vi "Pickle.vi"(0 "variant":variant) -> (4 "pickle":string)   [LabVIEW 2015, in "LV Exceptions v1.lvlib"]
doc: "Alternative to 'Variant To Flattened String' function. The advantages are:\n* it returns only printable characters\n* complimentary function doesn't need 'type string' argument"
uses:
  LV Exceptions v1.lvlib
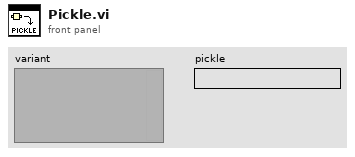
[diagram p1: front panel]
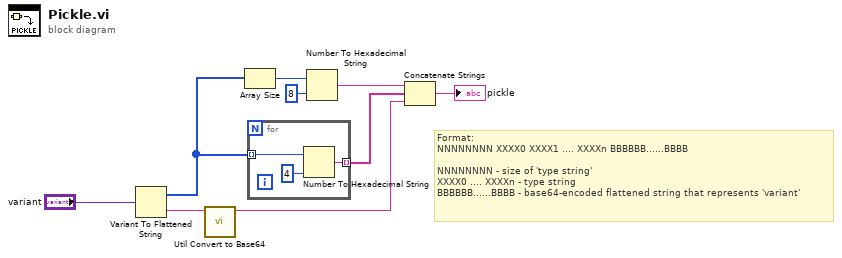
[diagram p0: block diagram]
diagram:
  # "Format:\nNNNNNNNN XXXX0 XXXX1 .... XXXXn BBBBBB......BBBB\n\nNNNNNNNN - size of 'type string'\nXXXX0 .... XXXXn - type string\nBBBBBB......BBBB - base64-encoded flattened string that represents 'variant'"
  n1 = Variant To Flattened String(Variant="variant") -> (data string=w9:string, 1:w6:i16[])
  n2 = call "Util Convert to Base64.vi"("String"=w9) -> ("Base64 String"=w3:string)  [unwired: 10 in]
  n3 = Array Size(array=w6) -> (size(s)=w8:i32)
  n4 = for {
    tunnel: w6 -> [w12] mode=indexing
    tunnel: [w10] -> w4 mode=indexing
    n5 = Number To Hexadecimal String(1:i16 4 ("width (-)"), 2:w12) -> (0:w10:string)
  }
  n6 = Number To Hexadecimal String(1:i16 8 ("width (-)"), 2:w8) -> (0:w5:string)
  n7 = Concatenate Strings(w5, w4, w3) -> (→"pickle":string)
